vi "Main.vi"() -> ()   [LabVIEW 2021] (continued)
                    w1503 = T9 27 items=["刷新间隔", "波特率", "布尔1设置项", "布尔2设置项", "布尔3设置项", "布尔4设置项", "布尔5设置项", "布尔6设置项", "布尔7设置项", "布尔8设置项", "显控1设置", "显控2设置", "显控3设置", "显控4设置", "显控5设置", "显控6设置", "显控7设置", "显控8设置", "显控9设置", "显控10设置", "显控11设置", "显控12设置", "设控1设置", "设控2设置", "设控3设置", "设控4设置", "设控5设置", "设控6设置", "设控7设置", "设控8设置", "曲线1设置", "曲线2设置", "曲线3设置", "曲线4设置", "曲线5设置", "曲线6设置", "曲线7设置", "曲线8设置", "曲线9设置", "曲线10设置", "曲线11设置", "曲线12设置", "曲线13设置", "曲线14设置", "曲线15设置", "曲线16设置", "曲线17设置", "曲线18设置", "曲线19设置", "曲线20设置", "曲线21设置", "曲线22设置", "曲线23设置", "曲线24设置", "曲线25设置", "曲线26设置", "曲线27设置", "曲线28设置", "曲线29设置", "曲线30设置", "曲线31设置", "曲线32设置", "曲线33设置", "曲线34设置", "曲线35设置", "曲线36设置", "曲线37设置", "曲线38设置", "曲线39设置", "曲线40设置", "曲线41设置", "曲线42设置", "曲线43设置", "曲线44设置", "曲线45设置", "曲线46设置", "曲线47设置", "曲线48设置", "曲线49设置", "曲线50设置", "曲线51设置", "曲线52设置", "曲线53设置", "曲线54设置", "曲线55设置", "曲线56设置", "曲线57设置", "曲线58设置", "曲线59设置", "曲线60设置", "曲线61设置", "曲线62设置", "曲线63设置", "曲线64设置", "ID值", "数据模式"] ("DataInitDef")
                    n1213 = property on="表格" class="Tbl (严格)"() -> ("Selection Start"=w1510:T1)  [unwired: 2 in, 2 out]
                    n1214 = Unbundle By Name(w1510) -> ("Row"=w1512:i32)
                    n1215 = property on="表格" class="Tbl (严格)"() -> ("Value"=w1511:string[][])  [unwired: 2 in, 2 out]
                    n1216 = Number To Decimal String(number=w1512) -> (decimal integer string=w1513:string)  [unwired: 1 in]
                    n1217 = Index Array(array=w1511, index (row)=w1512, index (col)=0 ("禁用的索引 (列)")) -> (element=w1505:string)
                    n1218 = String Subset(string=w1505, length (rest)=16 ("长度（剩余）")) -> (substring=w1504:string)  [unwired: 1 in]
                    n1219 = invoke on="控件配置文件" class="Tbl (严格)" method="Set Cell Value"("X Index"=1 ("X索引"), "Y Index"=w1503, "Value"=w1513) -> ()  [unwired: 3 in, 6 out]
                    n1220 = property on="设控6" class="Str"("Caption.Text"=w1504) -> ()  [unwired: 2 in, 2 out]
                    n1221 = property on="设控设置 6" class="Str"("Val(Sgnl)"=w1504) -> ()  [unwired: 2 in, 2 out]
                    n1222 = invoke on="控件配置文件" class="Tbl (严格)" method="Set Cell Value"("X Index"=0 ("X索引"), "Y Index"=w1503, "Value"=w1504) -> ()  [unwired: 3 in, 6 out]
                  }
                  frame "关联到设控7" {
                    w1514 = T9 28 items=["刷新间隔", "波特率", "布尔1设置项", "布尔2设置项", "布尔3设置项", "布尔4设置项", "布尔5设置项", "布尔6设置项", "布尔7设置项", "布尔8设置项", "显控1设置", "显控2设置", "显控3设置", "显控4设置", "显控5设置", "显控6设置", "显控7设置", "显控8设置", "显控9设置", "显控10设置", "显控11设置", "显控12设置", "设控1设置", "设控2设置", "设控3设置", "设控4设置", "设控5设置", "设控6设置", "设控7设置", "设控8设置", "曲线1设置", "曲线2设置", "曲线3设置", "曲线4设置", "曲线5设置", "曲线6设置", "曲线7设置", "曲线8设置", "曲线9设置", "曲线10设置", "曲线11设置", "曲线12设置", "曲线13设置", "曲线14设置", "曲线15设置", "曲线16设置", "曲线17设置", "曲线18设置", "曲线19设置", "曲线20设置", "曲线21设置", "曲线22设置", "曲线23设置", "曲线24设置", "曲线25设置", "曲线26设置", "曲线27设置", "曲线28设置", "曲线29设置", "曲线30设置", "曲线31设置", "曲线32设置", "曲线33设置", "曲线34设置", "曲线35设置", "曲线36设置", "曲线37设置", "曲线38设置", "曲线39设置", "曲线40设置", "曲线41设置", "曲线42设置", "曲线43设置", "曲线44设置", "曲线45设置", "曲线46设置", "曲线47设置", "曲线48设置", "曲线49设置", "曲线50设置", "曲线51设置", "曲线52设置", "曲线53设置", "曲线54设置", "曲线55设置", "曲线56设置", "曲线57设置", "曲线58设置", "曲线59设置", "曲线60设置", "曲线61设置", "曲线62设置", "曲线63设置", "曲线64设置", "ID值", "数据模式"] ("DataInitDef")
                    n1223 = property on="表格" class="Tbl (严格)"() -> ("Selection Start"=w1524:T1)  [unwired: 2 in, 2 out]
                    n1224 = Unbundle By Name(w1524) -> ("Row"=w1522:i32)
                    n1225 = property on="表格" class="Tbl (严格)"() -> ("Value"=w1523:string[][])  [unwired: 2 in, 2 out]
                    n1226 = Number To Decimal String(number=w1522) -> (decimal integer string=w1521:string)  [unwired: 1 in]
                    n1227 = Index Array(array=w1523, index (row)=w1522, index (col)=0 ("禁用的索引 (列)")) -> (element=w1516:string)
                    n1228 = String Subset(string=w1516, length (rest)=16 ("长度（剩余）")) -> (substring=w1515:string)  [unwired: 1 in]
                    n1229 = invoke on="控件配置文件" class="Tbl (严格)" method="Set Cell Value"("X Index"=1 ("X索引"), "Y Index"=w1514, "Value"=w1521) -> ()  [unwired: 3 in, 6 out]
                    n1230 = property on="设控7" class="Str"("Caption.Text"=w1515) -> ()  [unwired: 2 in, 2 out]
                    n1231 = property on="设控设置 7" class="Str"("Val(Sgnl)"=w1515) -> ()  [unwired: 2 in, 2 out]
                    n1232 = invoke on="控件配置文件" class="Tbl (严格)" method="Set Cell Value"("X Index"=0 ("X索引"), "Y Index"=w1514, "Value"=w1515) -> ()  [unwired: 3 in, 6 out]
                  }
                  frame "关联到设控8" {
                    w1525 = T9 29 items=["刷新间隔", "波特率", "布尔1设置项", "布尔2设置项", "布尔3设置项", "布尔4设置项", "布尔5设置项", "布尔6设置项", "布尔7设置项", "布尔8设置项", "显控1设置", "显控2设置", "显控3设置", "显控4设置", "显控5设置", "显控6设置", "显控7设置", "显控8设置", "显控9设置", "显控10设置", "显控11设置", "显控12设置", "设控1设置", "设控2设置", "设控3设置", "设控4设置", "设控5设置", "设控6设置", "设控7设置", "设控8设置", "曲线1设置", "曲线2设置", "曲线3设置", "曲线4设置", "曲线5设置", "曲线6设置", "曲线7设置", "曲线8设置", "曲线9设置", "曲线10设置", "曲线11设置", "曲线12设置", "曲线13设置", "曲线14设置", "曲线15设置", "曲线16设置", "曲线17设置", "曲线18设置", "曲线19设置", "曲线20设置", "曲线21设置", "曲线22设置", "曲线23设置", "曲线24设置", "曲线25设置", "曲线26设置", "曲线27设置", "曲线28设置", "曲线29设置", "曲线30设置", "曲线31设置", "曲线32设置", "曲线33设置", "曲线34设置", "曲线35设置", "曲线36设置", "曲线37设置", "曲线38设置", "曲线39设置", "曲线40设置", "曲线41设置", "曲线42设置", "曲线43设置", "曲线44设置", "曲线45设置", "曲线46设置", "曲线47设置", "曲线48设置", "曲线49设置", "曲线50设置", "曲线51设置", "曲线52设置", "曲线53设置", "曲线54设置", "曲线55设置", "曲线56设置", "曲线57设置", "曲线58设置", "曲线59设置", "曲线60设置", "曲线61设置", "曲线62设置", "曲线63设置", "曲线64设置", "ID值", "数据模式"] ("DataInitDef")
                    n1233 = property on="表格" class="Tbl (严格)"() -> ("Selection Start"=w1532:T1)  [unwired: 2 in, 2 out]
                    n1234 = Unbundle By Name(w1532) -> ("Row"=w1534:i32)
                    n1235 = property on="表格" class="Tbl (严格)"() -> ("Value"=w1533:string[][])  [unwired: 2 in, 2 out]
                    n1236 = Number To Decimal String(number=w1534) -> (decimal integer string=w1535:string)  [unwired: 1 in]
                    n1237 = Index Array(array=w1533, index (row)=w1534, index (col)=0 ("禁用的索引 (列)")) -> (element=w1527:string)
                    n1238 = String Subset(string=w1527, length (rest)=16 ("长度（剩余）")) -> (substring=w1526:string)  [unwired: 1 in]
                    n1239 = invoke on="控件配置文件" class="Tbl (严格)" method="Set Cell Value"("X Index"=1 ("X索引"), "Y Index"=w1525, "Value"=w1535) -> ()  [unwired: 3 in, 6 out]
                    n1240 = property on="设控8" class="Str"("Caption.Text"=w1526) -> ()  [unwired: 2 in, 2 out]
                    n1241 = property on="设控设置 8" class="Str"("Val(Sgnl)"=w1526) -> ()  [unwired: 2 in, 2 out]
                    n1242 = invoke on="控件配置文件" class="Tbl (严格)" method="Set Cell Value"("X Index"=0 ("X索引"), "Y Index"=w1525, "Value"=w1526) -> ()  [unwired: 3 in, 6 out]
                  }
                }
              }
            }
          }
          frame #2 {
            # "快捷菜单激活何批量EEPROM、数据导出"
            n1243 = event shown="[1] 菜单选择(用户);  \"表格\": 快捷菜单选择（用户）" {
              selector: _ -> [_ _]
              dyn-events: _ -> [_ _]
              timeout: 0 -> [_ _]
              event Timeout {
                n1244 = event-data() -> ()  [unwired: 1 in, 3 out]
              }
              event Menu Selection (User); "表格": Shortcut Menu Selection (User) {
                n1245 = event-data() -> ("ItemTag"=w1549:string)  [unwired: 1 in, 5 out]
                n1246 = case shown="\"批量写入EEPROM\"" w1549 {
                  frame "假", Default {
                  }
                  frame "导出参数" {
                    n1247 = property on="表格" class="Tbl (严格)"() -> ("Value"=w1552:string[][])  [unwired: 2 in, 2 out]
                    n1248 = call <vilib>:"Application Directory.vi"() -> ("Application Directory"=w1551:path)
                    n1249 = call "导出参数.vi"("名称或相对路径"="Config\\导出参数列表.xltx", "基路径"=w1551, "表格控件"=w1552) -> ()  [unwired: 9 in]
                  }
                  frame "批量写入EEPROM" {
                    n1250 = local read "刷新间隔"() -> (w1559:string)
                    n1251 = Decimal String To Number(string=w1559) -> (number=w1557:i32)  [unwired: 2 in, 1 out]
                    n1252 = local read "CAN通道"() -> (w1553:u8)
                    n1253 = local read "ID"() -> (w1554:u32)
                    n1254 = Less Or Equal?(x=w1557, y=1) -> (x <= y?=w1555:bool)
                    n1255 = Select(t=1, s=w1555, f=w1557) -> (s? t:f=w1558:i32)
                    n1256 = call "批量写入EEPROM.vi"("等待时间（毫秒）"=w1558, "ID"=w1554, "CAN通道"=w1553) -> ()  [unwired: 8 in]
                  }
                }
              }
            }
            n1257 = event shown="[1] \"波形图表\": 快捷菜单激活？" {
              selector: _ -> [_ _]
              dyn-events: _ -> [_ _]
              timeout: 0 -> [_ _]
              event Timeout {
                n1258 = event-data() -> ()  [unwired: 1 in, 3 out]
              }
              event "波形图表": Shortcut Menu Activation? {
                n1259 = event-data() -> ("MenuRef"=w1548:refnum<k9>)  [unwired: 1 in]
                n1260 = call "快捷菜单激活(波形图表).vi"("菜单引用"=w1548) -> ()  [unwired: 11 in]
                n1261 = event-data() -> ()  [unwired: 2 in, 1 out]
              }
            }
            n1262 = event shown="[1] \"表格\": 快捷菜单激活？" {
              selector: _ -> [_ _]
              dyn-events: _ -> [_ _]
              timeout: 0 -> [_ _]
              event Timeout {
                n1263 = event-data() -> ()  [unwired: 1 in, 3 out]
              }
              event "表格": Shortcut Menu Activation? {
                # "激活表格右击菜单选项"
                n1264 = event-data() -> ("MenuRef"=w1561:refnum<k9>)  [unwired: 1 in]
                n1265 = call "快捷菜单激活(表格).vi"("菜单引用"=w1561) -> ()  [unwired: 11 in]
                n1266 = event-data() -> ()  [unwired: 2 in, 1 out]
              }
            }
            n1267 = event shown="[1] \"布尔 1\", \"布尔 2\", \"布尔 3\", \"布尔 4\", \"布尔 5\", \"布尔 6\", \"布尔 7\", \"布尔 8\": 快捷菜单激活？" {
              selector: _ -> [_ _ _ _ _]
              dyn-events: _ -> [_ _ _ _ _]
              timeout: 0 -> [_ _ _ _ _]
              event Timeout {
                n1268 = event-data() -> ()  [unwired: 1 in, 3 out]
              }
              event "布尔 1", "布尔 2", "布尔 3", "布尔 4", "布尔 5", "布尔 6", "布尔 7", "布尔 8": Shortcut Menu Activation? {
                # "撤销布尔控件的关联"
                n1269 = event-data() -> ("MenuRef"=w1541:refnum<k9>)  [unwired: 1 in, 3 out]
                n1270 = Insert Menu Items(8:string[] ["撤销关联"] ("项名称"), 9:w1541) -> ()  [unwired: 4 in, 3 out]
                n1271 = event-data() -> ()  [unwired: 2 in, 1 out]
              }
              event "显控1", "显控6", "显控7", "显控2", "显控3", "显控4", "显控8", "显控9", "显控10", "显控11", "显控12", "显控5": Shortcut Menu Activation? {
                n1272 = event-data() -> ("MenuRef"=w1542:refnum<k9>)  [unwired: 1 in, 4 out]
                n1273 = Insert Menu Items(8:string[] ["撤销关联"] ("项名称"), 9:w1542) -> ()  [unwired: 4 in, 3 out]
                n1274 = event-data() -> ()  [unwired: 2 in, 1 out]
              }
              event "设控1", "设控2", "设控3", "设控4", "设控5", "设控6", "设控7", "设控8": Shortcut Menu Activation? {
                n1275 = event-data() -> ("MenuRef"=w1544:refnum<k9>)  [unwired: 1 in, 5 out]
                n1276 = event-data() -> ()  [unwired: 2 in, 1 out]
                n1277 = Insert Menu Items(8:string[] ["撤销关联"] ("项名称"), 9:w1544) -> ()  [unwired: 4 in, 3 out]
              }
              event "状态显示": Shortcut Menu Activation? {
                n1278 = event-data() -> ("MenuRef"=w1546:refnum<k9>)  [unwired: 1 in, 5 out]
                n1279 = event-data() -> ()  [unwired: 2 in, 1 out]
                n1280 = Insert Menu Items(8:string[] ["撤销关联"] ("项名称"), 9:w1546) -> ()  [unwired: 4 in, 3 out]
              }
            }
          }
          frame #3 {
            # "所有控件撤销关联代码"
            n1281 = event shown="[21] \"波形图表\": 快捷菜单选择（用户）" {
              selector: _ -> [_ _ _ _ _ _ _ _ _ _ _ _ _ _ _ _ _ _ _ _ _ _ _ _ _ _ _ _ _ _]
              dyn-events: _ -> [_ _ _ _ _ _ _ _ _ _ _ _ _ _ _ _ _ _ _ _ _ _ _ _ _ _ _ _ _ _]
              timeout: 0 -> [_ _ _ _ _ _ _ _ _ _ _ _ _ _ _ _ _ _ _ _ _ _ _ _ _ _ _ _ _ _]
              event Timeout {
                n1282 = event-data() -> ()  [unwired: 1 in, 3 out]
              }
              event "布尔 1": Shortcut Menu Selection (User) {
                w1563 = T9 2 items=["刷新间隔", "波特率", "布尔1设置项", "布尔2设置项", "布尔3设置项", "布尔4设置项", "布尔5设置项", "布尔6设置项", "布尔7设置项", "布尔8设置项", "显控1设置", "显控2设置", "显控3设置", "显控4设置", "显控5设置", "显控6设置", "显控7设置", "显控8设置", "显控9设置", "显控10设置", "显控11设置", "显控12设置", "设控1设置", "设控2设置", "设控3设置", "设控4设置", "设控5设置", "设控6设置", "设控7设置", "设控8设置", "曲线1设置", "曲线2设置", "曲线3设置", "曲线4设置", "曲线5设置", "曲线6设置", "曲线7设置", "曲线8设置", "曲线9设置", "曲线10设置", "曲线11设置", "曲线12设置", "曲线13设置", "曲线14设置", "曲线15设置", "曲线16设置", "曲线17设置", "曲线18设置", "曲线19设置", "曲线20设置", "曲线21设置", "曲线22设置", "曲线23设置", "曲线24设置", "曲线25设置", "曲线26设置", "曲线27设置", "曲线28设置", "曲线29设置", "曲线30设置", "曲线31设置", "曲线32设置", "曲线33设置", "曲线34设置", "曲线35设置", "曲线36设置", "曲线37设置", "曲线38设置", "曲线39设置", "曲线40设置", "曲线41设置", "曲线42设置", "曲线43设置", "曲线44设置", "曲线45设置", "曲线46设置", "曲线47设置", "曲线48设置", "曲线49设置", "曲线50设置", "曲线51设置", "曲线52设置", "曲线53设置", "曲线54设置", "曲线55设置", "曲线56设置", "曲线57设置", "曲线58设置", "曲线59设置", "曲线60设置", "曲线61设置", "曲线62设置", "曲线63设置", "曲线64设置", "ID值", "数据模式"] ("DataInitDef")
                w1564 = "布尔 1" ("标题.文本")
                # "撤销关联的代码"
                n1283 = event-data() -> ()  [unwired: 1 in, 8 out]
                n1284 = invoke on="控件配置文件" class="Tbl (严格)" method="Set Cell Value"("X Index"=1 ("X索引"), "Y Index"=w1563, "Value"="X" ("值")) -> ()  [unwired: 3 in, 6 out]
                n1285 = invoke on="控件配置文件" class="Tbl (严格)" method="Set Cell Value"("X Index"=0 ("X索引"), "Y Index"=w1563, "Value"=w1564) -> ()  [unwired: 3 in, 6 out]
                n1286 = property on="布尔 1" class="Bool (严格)"("Caption.Text"=w1564) -> ()  [unwired: 2 in, 2 out]
                n1287 = property on="布控1设置" class="Str"("Val(Sgnl)"=w1564) -> ()  [unwired: 2 in, 2 out]
              }
              event "布尔 2": Shortcut Menu Selection (User) {
                w1568 = T9 3 items=["刷新间隔", "波特率", "布尔1设置项", "布尔2设置项", "布尔3设置项", "布尔4设置项", "布尔5设置项", "布尔6设置项", "布尔7设置项", "布尔8设置项", "显控1设置", "显控2设置", "显控3设置", "显控4设置", "显控5设置", "显控6设置", "显控7设置", "显控8设置", "显控9设置", "显控10设置", "显控11设置", "显控12设置", "设控1设置", "设控2设置", "设控3设置", "设控4设置", "设控5设置", "设控6设置", "设控7设置", "设控8设置", "曲线1设置", "曲线2设置", "曲线3设置", "曲线4设置", "曲线5设置", "曲线6设置", "曲线7设置", "曲线8设置", "曲线9设置", "曲线10设置", "曲线11设置", "曲线12设置", "曲线13设置", "曲线14设置", "曲线15设置", "曲线16设置", "曲线17设置", "曲线18设置", "曲线19设置", "曲线20设置", "曲线21设置", "曲线22设置", "曲线23设置", "曲线24设置", "曲线25设置", "曲线26设置", "曲线27设置", "曲线28设置", "曲线29设置", "曲线30设置", "曲线31设置", "曲线32设置", "曲线33设置", "曲线34设置", "曲线35设置", "曲线36设置", "曲线37设置", "曲线38设置", "曲线39设置", "曲线40设置", "曲线41设置", "曲线42设置", "曲线43设置", "曲线44设置", "曲线45设置", "曲线46设置", "曲线47设置", "曲线48设置", "曲线49设置", "曲线50设置", "曲线51设置", "曲线52设置", "曲线53设置", "曲线54设置", "曲线55设置", "曲线56设置", "曲线57设置", "曲线58设置", "曲线59设置", "曲线60设置", "曲线61设置", "曲线62设置", "曲线63设置", "曲线64设置", "ID值", "数据模式"] ("DataInitDef")
                w1569 = "布尔 2" ("标题.文本")
                n1288 = event-data() -> ()  [unwired: 1 in, 8 out]
                n1289 = invoke on="控件配置文件" class="Tbl (严格)" method="Set Cell Value"("X Index"=1 ("X索引"), "Y Index"=w1568, "Value"="X" ("值")) -> ()  [unwired: 3 in, 6 out]
                n1290 = invoke on="控件配置文件" class="Tbl (严格)" method="Set Cell Value"("X Index"=0 ("X索引"), "Y Index"=w1568, "Value"=w1569) -> ()  [unwired: 3 in, 6 out]
                n1291 = property on="布控2设置" class="Str"("Val(Sgnl)"=w1569) -> ()  [unwired: 2 in, 2 out]
                n1292 = property on="布尔 2" class="Bool (严格)"("Caption.Text"=w1569) -> ()  [unwired: 2 in, 2 out]
              }
              event "布尔 3": Shortcut Menu Selection (User) {
                w1573 = T9 4 items=["刷新间隔", "波特率", "布尔1设置项", "布尔2设置项", "布尔3设置项", "布尔4设置项", "布尔5设置项", "布尔6设置项", "布尔7设置项", "布尔8设置项", "显控1设置", "显控2设置", "显控3设置", "显控4设置", "显控5设置", "显控6设置", "显控7设置", "显控8设置", "显控9设置", "显控10设置", "显控11设置", "显控12设置", "设控1设置", "设控2设置", "设控3设置", "设控4设置", "设控5设置", "设控6设置", "设控7设置", "设控8设置", "曲线1设置", "曲线2设置", "曲线3设置", "曲线4设置", "曲线5设置", "曲线6设置", "曲线7设置", "曲线8设置", "曲线9设置", "曲线10设置", "曲线11设置", "曲线12设置", "曲线13设置", "曲线14设置", "曲线15设置", "曲线16设置", "曲线17设置", "曲线18设置", "曲线19设置", "曲线20设置", "曲线21设置", "曲线22设置", "曲线23设置", "曲线24设置", "曲线25设置", "曲线26设置", "曲线27设置", "曲线28设置", "曲线29设置", "曲线30设置", "曲线31设置", "曲线32设置", "曲线33设置", "曲线34设置", "曲线35设置", "曲线36设置", "曲线37设置", "曲线38设置", "曲线39设置", "曲线40设置", "曲线41设置", "曲线42设置", "曲线43设置", "曲线44设置", "曲线45设置", "曲线46设置", "曲线47设置", "曲线48设置", "曲线49设置", "曲线50设置", "曲线51设置", "曲线52设置", "曲线53设置", "曲线54设置", "曲线55设置", "曲线56设置", "曲线57设置", "曲线58设置", "曲线59设置", "曲线60设置", "曲线61设置", "曲线62设置", "曲线63设置", "曲线64设置", "ID值", "数据模式"] ("DataInitDef")
                w1574 = "布尔 3" ("标题.文本")
                n1293 = event-data() -> ()  [unwired: 1 in, 8 out]
                n1294 = invoke on="控件配置文件" class="Tbl (严格)" method="Set Cell Value"("X Index"=1 ("X索引"), "Y Index"=w1573, "Value"="X" ("值")) -> ()  [unwired: 3 in, 6 out]
                n1295 = invoke on="控件配置文件" class="Tbl (严格)" method="Set Cell Value"("X Index"=0 ("X索引"), "Y Index"=w1573, "Value"=w1574) -> ()  [unwired: 3 in, 6 out]
                n1296 = property on="布尔 3" class="Bool (严格)"("Caption.Text"=w1574) -> ()  [unwired: 2 in, 2 out]
                n1297 = property on="布控3设置" class="Str"("Val(Sgnl)"=w1574) -> ()  [unwired: 2 in, 2 out]
              }
              event "布尔 4": Shortcut Menu Selection (User) {
                w1578 = T9 5 items=["刷新间隔", "波特率", "布尔1设置项", "布尔2设置项", "布尔3设置项", "布尔4设置项", "布尔5设置项", "布尔6设置项", "布尔7设置项", "布尔8设置项", "显控1设置", "显控2设置", "显控3设置", "显控4设置", "显控5设置", "显控6设置", "显控7设置", "显控8设置", "显控9设置", "显控10设置", "显控11设置", "显控12设置", "设控1设置", "设控2设置", "设控3设置", "设控4设置", "设控5设置", "设控6设置", "设控7设置", "设控8设置", "曲线1设置", "曲线2设置", "曲线3设置", "曲线4设置", "曲线5设置", "曲线6设置", "曲线7设置", "曲线8设置", "曲线9设置", "曲线10设置", "曲线11设置", "曲线12设置", "曲线13设置", "曲线14设置", "曲线15设置", "曲线16设置", "曲线17设置", "曲线18设置", "曲线19设置", "曲线20设置", "曲线21设置", "曲线22设置", "曲线23设置", "曲线24设置", "曲线25设置", "曲线26设置", "曲线27设置", "曲线28设置", "曲线29设置", "曲线30设置", "曲线31设置", "曲线32设置", "曲线33设置", "曲线34设置", "曲线35设置", "曲线36设置", "曲线37设置", "曲线38设置", "曲线39设置", "曲线40设置", "曲线41设置", "曲线42设置", "曲线43设置", "曲线44设置", "曲线45设置", "曲线46设置", "曲线47设置", "曲线48设置", "曲线49设置", "曲线50设置", "曲线51设置", "曲线52设置", "曲线53设置", "曲线54设置", "曲线55设置", "曲线56设置", "曲线57设置", "曲线58设置", "曲线59设置", "曲线60设置", "曲线61设置", "曲线62设置", "曲线63设置", "曲线64设置", "ID值", "数据模式"] ("DataInitDef")
                w1579 = "布尔 4" ("标题.文本")
                n1298 = event-data() -> ()  [unwired: 1 in, 8 out]
                n1299 = invoke on="控件配置文件" class="Tbl (严格)" method="Set Cell Value"("X Index"=1 ("X索引"), "Y Index"=w1578, "Value"="X" ("值")) -> ()  [unwired: 3 in, 6 out]
                n1300 = invoke on="控件配置文件" class="Tbl (严格)" method="Set Cell Value"("X Index"=0 ("X索引"), "Y Index"=w1578, "Value"=w1579) -> ()  [unwired: 3 in, 6 out]
                n1301 = property on="布尔 4" class="Bool (严格)"("Caption.Text"=w1579) -> ()  [unwired: 2 in, 2 out]
                n1302 = property on="布控4设置" class="Str"("Val(Sgnl)"=w1579) -> ()  [unwired: 2 in, 2 out]
              }
              event "布尔 5": Shortcut Menu Selection (User) {
                w1583 = T9 6 items=["刷新间隔", "波特率", "布尔1设置项", "布尔2设置项", "布尔3设置项", "布尔4设置项", "布尔5设置项", "布尔6设置项", "布尔7设置项", "布尔8设置项", "显控1设置", "显控2设置", "显控3设置", "显控4设置", "显控5设置", "显控6设置", "显控7设置", "显控8设置", "显控9设置", "显控10设置", "显控11设置", "显控12设置", "设控1设置", "设控2设置", "设控3设置", "设控4设置", "设控5设置", "设控6设置", "设控7设置", "设控8设置", "曲线1设置", "曲线2设置", "曲线3设置", "曲线4设置", "曲线5设置", "曲线6设置", "曲线7设置", "曲线8设置", "曲线9设置", "曲线10设置", "曲线11设置", "曲线12设置", "曲线13设置", "曲线14设置", "曲线15设置", "曲线16设置", "曲线17设置", "曲线18设置", "曲线19设置", "曲线20设置", "曲线21设置", "曲线22设置", "曲线23设置", "曲线24设置", "曲线25设置", "曲线26设置", "曲线27设置", "曲线28设置", "曲线29设置", "曲线30设置", "曲线31设置", "曲线32设置", "曲线33设置", "曲线34设置", "曲线35设置", "曲线36设置", "曲线37设置", "曲线38设置", "曲线39设置", "曲线40设置", "曲线41设置", "曲线42设置", "曲线43设置", "曲线44设置", "曲线45设置", "曲线46设置", "曲线47设置", "曲线48设置", "曲线49设置", "曲线50设置", "曲线51设置", "曲线52设置", "曲线53设置", "曲线54设置", "曲线55设置", "曲线56设置", "曲线57设置", "曲线58设置", "曲线59设置", "曲线60设置", "曲线61设置", "曲线62设置", "曲线63设置", "曲线64设置", "ID值", "数据模式"] ("DataInitDef")
                w1587 = "布尔 5" ("标题.文本")
                n1303 = event-data() -> ()  [unwired: 1 in, 8 out]
                n1304 = invoke on="控件配置文件" class="Tbl (严格)" method="Set Cell Value"("X Index"=1 ("X索引"), "Y Index"=w1583, "Value"="X" ("值")) -> ()  [unwired: 3 in, 6 out]
                n1305 = invoke on="控件配置文件" class="Tbl (严格)" method="Set Cell Value"("X Index"=0 ("X索引"), "Y Index"=w1583, "Value"=w1587) -> ()  [unwired: 3 in, 6 out]
                n1306 = property on="布尔 5" class="Bool (严格)"("Caption.Text"=w1587) -> ()  [unwired: 2 in, 2 out]
                n1307 = property on="布控5设置" class="Str"("Val(Sgnl)"=w1587) -> ()  [unwired: 2 in, 2 out]
              }
              event "布尔 6": Shortcut Menu Selection (User) {
                w1590 = T9 7 items=["刷新间隔", "波特率", "布尔1设置项", "布尔2设置项", "布尔3设置项", "布尔4设置项", "布尔5设置项", "布尔6设置项", "布尔7设置项", "布尔8设置项", "显控1设置", "显控2设置", "显控3设置", "显控4设置", "显控5设置", "显控6设置", "显控7设置", "显控8设置", "显控9设置", "显控10设置", "显控11设置", "显控12设置", "设控1设置", "设控2设置", "设控3设置", "设控4设置", "设控5设置", "设控6设置", "设控7设置", "设控8设置", "曲线1设置", "曲线2设置", "曲线3设置", "曲线4设置", "曲线5设置", "曲线6设置", "曲线7设置", "曲线8设置", "曲线9设置", "曲线10设置", "曲线11设置", "曲线12设置", "曲线13设置", "曲线14设置", "曲线15设置", "曲线16设置", "曲线17设置", "曲线18设置", "曲线19设置", "曲线20设置", "曲线21设置", "曲线22设置", "曲线23设置", "曲线24设置", "曲线25设置", "曲线26设置", "曲线27设置", "曲线28设置", "曲线29设置", "曲线30设置", "曲线31设置", "曲线32设置", "曲线33设置", "曲线34设置", "曲线35设置", "曲线36设置", "曲线37设置", "曲线38设置", "曲线39设置", "曲线40设置", "曲线41设置", "曲线42设置", "曲线43设置", "曲线44设置", "曲线45设置", "曲线46设置", "曲线47设置", "曲线48设置", "曲线49设置", "曲线50设置", "曲线51设置", "曲线52设置", "曲线53设置", "曲线54设置", "曲线55设置", "曲线56设置", "曲线57设置", "曲线58设置", "曲线59设置", "曲线60设置", "曲线61设置", "曲线62设置", "曲线63设置", "曲线64设置", "ID值", "数据模式"] ("DataInitDef")
                w1592 = "布尔 6" ("标题.文本")
                n1308 = event-data() -> ()  [unwired: 1 in, 8 out]
                n1309 = invoke on="控件配置文件" class="Tbl (严格)" method="Set Cell Value"("X Index"=1 ("X索引"), "Y Index"=w1590, "Value"="X" ("值")) -> ()  [unwired: 3 in, 6 out]
                n1310 = invoke on="控件配置文件" class="Tbl (严格)" method="Set Cell Value"("X Index"=0 ("X索引"), "Y Index"=w1590, "Value"=w1592) -> ()  [unwired: 3 in, 6 out]
                n1311 = property on="布尔 6" class="Bool (严格)"("Caption.Text"=w1592) -> ()  [unwired: 2 in, 2 out]
                n1312 = property on="布控6设置" class="Str"("Val(Sgnl)"=w1592) -> ()  [unwired: 2 in, 2 out]
              }
              event "布尔 7": Shortcut Menu Selection (User) {
                w1595 = T9 8 items=["刷新间隔", "波特率", "布尔1设置项", "布尔2设置项", "布尔3设置项", "布尔4设置项", "布尔5设置项", "布尔6设置项", "布尔7设置项", "布尔8设置项", "显控1设置", "显控2设置", "显控3设置", "显控4设置", "显控5设置", "显控6设置", "显控7设置", "显控8设置", "显控9设置", "显控10设置", "显控11设置", "显控12设置", "设控1设置", "设控2设置", "设控3设置", "设控4设置", "设控5设置", "设控6设置", "设控7设置", "设控8设置", "曲线1设置", "曲线2设置", "曲线3设置", "曲线4设置", "曲线5设置", "曲线6设置", "曲线7设置", "曲线8设置", "曲线9设置", "曲线10设置", "曲线11设置", "曲线12设置", "曲线13设置", "曲线14设置", "曲线15设置", "曲线16设置", "曲线17设置", "曲线18设置", "曲线19设置", "曲线20设置", "曲线21设置", "曲线22设置", "曲线23设置", "曲线24设置", "曲线25设置", "曲线26设置", "曲线27设置", "曲线28设置", "曲线29设置", "曲线30设置", "曲线31设置", "曲线32设置", "曲线33设置", "曲线34设置", "曲线35设置", "曲线36设置", "曲线37设置", "曲线38设置", "曲线39设置", "曲线40设置", "曲线41设置", "曲线42设置", "曲线43设置", "曲线44设置", "曲线45设置", "曲线46设置", "曲线47设置", "曲线48设置", "曲线49设置", "曲线50设置", "曲线51设置", "曲线52设置", "曲线53设置", "曲线54设置", "曲线55设置", "曲线56设置", "曲线57设置", "曲线58设置", "曲线59设置", "曲线60设置", "曲线61设置", "曲线62设置", "曲线63设置", "曲线64设置", "ID值", "数据模式"] ("DataInitDef")
                w1597 = "布尔 7" ("标题.文本")
                n1313 = event-data() -> ()  [unwired: 1 in, 8 out]
                n1314 = invoke on="控件配置文件" class="Tbl (严格)" method="Set Cell Value"("X Index"=1 ("X索引"), "Y Index"=w1595, "Value"="X" ("值")) -> ()  [unwired: 3 in, 6 out]
                n1315 = invoke on="控件配置文件" class="Tbl (严格)" method="Set Cell Value"("X Index"=0 ("X索引"), "Y Index"=w1595, "Value"=w1597) -> ()  [unwired: 3 in, 6 out]
                n1316 = property on="布尔 7" class="Bool (严格)"("Caption.Text"=w1597) -> ()  [unwired: 2 in, 2 out]
                n1317 = property on="布控7设置" class="Str"("Val(Sgnl)"=w1597) -> ()  [unwired: 2 in, 2 out]
              }
              event "布尔 8": Shortcut Menu Selection (User) {
                w1600 = T9 9 items=["刷新间隔", "波特率", "布尔1设置项", "布尔2设置项", "布尔3设置项", "布尔4设置项", "布尔5设置项", "布尔6设置项", "布尔7设置项", "布尔8设置项", "显控1设置", "显控2设置", "显控3设置", "显控4设置", "显控5设置", "显控6设置", "显控7设置", "显控8设置", "显控9设置", "显控10设置", "显控11设置", "显控12设置", "设控1设置", "设控2设置", "设控3设置", "设控4设置", "设控5设置", "设控6设置", "设控7设置", "设控8设置", "曲线1设置", "曲线2设置", "曲线3设置", "曲线4设置", "曲线5设置", "曲线6设置", "曲线7设置", "曲线8设置", "曲线9设置", "曲线10设置", "曲线11设置", "曲线12设置", "曲线13设置", "曲线14设置", "曲线15设置", "曲线16设置", "曲线17设置", "曲线18设置", "曲线19设置", "曲线20设置", "曲线21设置", "曲线22设置", "曲线23设置", "曲线24设置", "曲线25设置", "曲线26设置", "曲线27设置", "曲线28设置", "曲线29设置", "曲线30设置", "曲线31设置", "曲线32设置", "曲线33设置", "曲线34设置", "曲线35设置", "曲线36设置", "曲线37设置", "曲线38设置", "曲线39设置", "曲线40设置", "曲线41设置", "曲线42设置", "曲线43设置", "曲线44设置", "曲线45设置", "曲线46设置", "曲线47设置", "曲线48设置", "曲线49设置", "曲线50设置", "曲线51设置", "曲线52设置", "曲线53设置", "曲线54设置", "曲线55设置", "曲线56设置", "曲线57设置", "曲线58设置", "曲线59设置", "曲线60设置", "曲线61设置", "曲线62设置", "曲线63设置", "曲线64设置", "ID值", "数据模式"] ("DataInitDef")
                w1602 = "布尔 8" ("标题.文本")
                n1318 = event-data() -> ()  [unwired: 1 in, 8 out]
                n1319 = invoke on="控件配置文件" class="Tbl (严格)" method="Set Cell Value"("X Index"=1 ("X索引"), "Y Index"=w1600, "Value"="X" ("值")) -> ()  [unwired: 3 in, 6 out]
                n1320 = invoke on="控件配置文件" class="Tbl (严格)" method="Set Cell Value"("X Index"=0 ("X索引"), "Y Index"=w1600, "Value"=w1602) -> ()  [unwired: 3 in, 6 out]
                n1321 = property on="布尔 8" class="Bool (严格)"("Caption.Text"=w1602) -> ()  [unwired: 2 in, 2 out]
                n1322 = property on="布控8设置" class="Str"("Val(Sgnl)"=w1602) -> ()  [unwired: 2 in, 2 out]
              }
              event "显控1": Shortcut Menu Selection (User) {
                w1603 = T9 10 items=["刷新间隔", "波特率", "布尔1设置项", "布尔2设置项", "布尔3设置项", "布尔4设置项", "布尔5设置项", "布尔6设置项", "布尔7设置项", "布尔8设置项", "显控1设置", "显控2设置", "显控3设置", "显控4设置", "显控5设置", "显控6设置", "显控7设置", "显控8设置", "显控9设置", "显控10设置", "显控11设置", "显控12设置", "设控1设置", "设控2设置", "设控3设置", "设控4设置", "设控5设置", "设控6设置", "设控7设置", "设控8设置", "曲线1设置", "曲线2设置", "曲线3设置", "曲线4设置", "曲线5设置", "曲线6设置", "曲线7设置", "曲线8设置", "曲线9设置", "曲线10设置", "曲线11设置", "曲线12设置", "曲线13设置", "曲线14设置", "曲线15设置", "曲线16设置", "曲线17设置", "曲线18设置", "曲线19设置", "曲线20设置", "曲线21设置", "曲线22设置", "曲线23设置", "曲线24设置", "曲线25设置", "曲线26设置", "曲线27设置", "曲线28设置", "曲线29设置", "曲线30设置", "曲线31设置", "曲线32设置", "曲线33设置", "曲线34设置", "曲线35设置", "曲线36设置", "曲线37设置", "曲线38设置", "曲线39设置", "曲线40设置", "曲线41设置", "曲线42设置", "曲线43设置", "曲线44设置", "曲线45设置", "曲线46设置", "曲线47设置", "曲线48设置", "曲线49设置", "曲线50设置", "曲线51设置", "曲线52设置", "曲线53设置", "曲线54设置", "曲线55设置", "曲线56设置", "曲线57设置", "曲线58设置", "曲线59设置", "曲线60设置", "曲线61设置", "曲线62设置", "曲线63设置", "曲线64设置", "ID值", "数据模式"] ("DataInitDef")
                w1604 = "显控1" ("标题.文本")
                # "撤销显控关联"
                n1323 = event-data() -> ()  [unwired: 1 in, 8 out]
                n1324 = invoke on="控件配置文件" class="Tbl (严格)" method="Set Cell Value"("X Index"=1 ("X索引"), "Y Index"=w1603, "Value"="X" ("值")) -> ()  [unwired: 3 in, 6 out]
                n1325 = invoke on="控件配置文件" class="Tbl (严格)" method="Set Cell Value"("X Index"=0 ("X索引"), "Y Index"=w1603, "Value"=w1604) -> ()  [unwired: 3 in, 6 out]
                n1326 = property on="显控1" class="Str"("Caption.Text"=w1604) -> ()  [unwired: 2 in, 2 out]
                n1327 = property on="显控1设置" class="Str"("Val(Sgnl)"=w1604) -> ()  [unwired: 2 in, 2 out]
              }
              event "显控2": Shortcut Menu Selection (User) {
                w1608 = T9 11 items=["刷新间隔", "波特率", "布尔1设置项", "布尔2设置项", "布尔3设置项", "布尔4设置项", "布尔5设置项", "布尔6设置项", "布尔7设置项", "布尔8设置项", "显控1设置", "显控2设置", "显控3设置", "显控4设置", "显控5设置", "显控6设置", "显控7设置", "显控8设置", "显控9设置", "显控10设置", "显控11设置", "显控12设置", "设控1设置", "设控2设置", "设控3设置", "设控4设置", "设控5设置", "设控6设置", "设控7设置", "设控8设置", "曲线1设置", "曲线2设置", "曲线3设置", "曲线4设置", "曲线5设置", "曲线6设置", "曲线7设置", "曲线8设置", "曲线9设置", "曲线10设置", "曲线11设置", "曲线12设置", "曲线13设置", "曲线14设置", "曲线15设置", "曲线16设置", "曲线17设置", "曲线18设置", "曲线19设置", "曲线20设置", "曲线21设置", "曲线22设置", "曲线23设置", "曲线24设置", "曲线25设置", "曲线26设置", "曲线27设置", "曲线28设置", "曲线29设置", "曲线30设置", "曲线31设置", "曲线32设置", "曲线33设置", "曲线34设置", "曲线35设置", "曲线36设置", "曲线37设置", "曲线38设置", "曲线39设置", "曲线40设置", "曲线41设置", "曲线42设置", "曲线43设置", "曲线44设置", "曲线45设置", "曲线46设置", "曲线47设置", "曲线48设置", "曲线49设置", "曲线50设置", "曲线51设置", "曲线52设置", "曲线53设置", "曲线54设置", "曲线55设置", "曲线56设置", "曲线57设置", "曲线58设置", "曲线59设置", "曲线60设置", "曲线61设置", "曲线62设置", "曲线63设置", "曲线64设置", "ID值", "数据模式"] ("DataInitDef")
                w1609 = "显控2" ("标题.文本")
                n1328 = event-data() -> ()  [unwired: 1 in, 8 out]
                n1329 = invoke on="控件配置文件" class="Tbl (严格)" method="Set Cell Value"("X Index"=1 ("X索引"), "Y Index"=w1608, "Value"="X" ("值")) -> ()  [unwired: 3 in, 6 out]
                n1330 = invoke on="控件配置文件" class="Tbl (严格)" method="Set Cell Value"("X Index"=0 ("X索引"), "Y Index"=w1608, "Value"=w1609) -> ()  [unwired: 3 in, 6 out]
                n1331 = property on="显控2" class="Str"("Caption.Text"=w1609) -> ()  [unwired: 2 in, 2 out]
                n1332 = property on="显控2设置" class="Str"("Val(Sgnl)"=w1609) -> ()  [unwired: 2 in, 2 out]
              }
              event "显控3": Shortcut Menu Selection (User) {
                w1613 = T9 12 items=["刷新间隔", "波特率", "布尔1设置项", "布尔2设置项", "布尔3设置项", "布尔4设置项", "布尔5设置项", "布尔6设置项", "布尔7设置项", "布尔8设置项", "显控1设置", "显控2设置", "显控3设置", "显控4设置", "显控5设置", "显控6设置", "显控7设置", "显控8设置", "显控9设置", "显控10设置", "显控11设置", "显控12设置", "设控1设置", "设控2设置", "设控3设置", "设控4设置", "设控5设置", "设控6设置", "设控7设置", "设控8设置", "曲线1设置", "曲线2设置", "曲线3设置", "曲线4设置", "曲线5设置", "曲线6设置", "曲线7设置", "曲线8设置", "曲线9设置", "曲线10设置", "曲线11设置", "曲线12设置", "曲线13设置", "曲线14设置", "曲线15设置", "曲线16设置", "曲线17设置", "曲线18设置", "曲线19设置", "曲线20设置", "曲线21设置", "曲线22设置", "曲线23设置", "曲线24设置", "曲线25设置", "曲线26设置", "曲线27设置", "曲线28设置", "曲线29设置", "曲线30设置", "曲线31设置", "曲线32设置", "曲线33设置", "曲线34设置", "曲线35设置", "曲线36设置", "曲线37设置", "曲线38设置", "曲线39设置", "曲线40设置", "曲线41设置", "曲线42设置", "曲线43设置", "曲线44设置", "曲线45设置", "曲线46设置", "曲线47设置", "曲线48设置", "曲线49设置", "曲线50设置", "曲线51设置", "曲线52设置", "曲线53设置", "曲线54设置", "曲线55设置", "曲线56设置", "曲线57设置", "曲线58设置", "曲线59设置", "曲线60设置", "曲线61设置", "曲线62设置", "曲线63设置", "曲线64设置", "ID值", "数据模式"] ("DataInitDef")
                w1614 = "显控3" ("标题.文本")
                n1333 = event-data() -> ()  [unwired: 1 in, 8 out]
                n1334 = invoke on="控件配置文件" class="Tbl (严格)" method="Set Cell Value"("X Index"=1 ("X索引"), "Y Index"=w1613, "Value"="X" ("值")) -> ()  [unwired: 3 in, 6 out]
                n1335 = invoke on="控件配置文件" class="Tbl (严格)" method="Set Cell Value"("X Index"=0 ("X索引"), "Y Index"=w1613, "Value"=w1614) -> ()  [unwired: 3 in, 6 out]
                n1336 = property on="显控3" class="Str"("Caption.Text"=w1614) -> ()  [unwired: 2 in, 2 out]
                n1337 = property on="显控3设置" class="Str"("Val(Sgnl)"=w1614) -> ()  [unwired: 2 in, 2 out]
              }
              event "显控4": Shortcut Menu Selection (User) {
                w1618 = T9 13 items=["刷新间隔", "波特率", "布尔1设置项", "布尔2设置项", "布尔3设置项", "布尔4设置项", "布尔5设置项", "布尔6设置项", "布尔7设置项", "布尔8设置项", "显控1设置", "显控2设置", "显控3设置", "显控4设置", "显控5设置", "显控6设置", "显控7设置", "显控8设置", "显控9设置", "显控10设置", "显控11设置", "显控12设置", "设控1设置", "设控2设置", "设控3设置", "设控4设置", "设控5设置", "设控6设置", "设控7设置", "设控8设置", "曲线1设置", "曲线2设置", "曲线3设置", "曲线4设置", "曲线5设置", "曲线6设置", "曲线7设置", "曲线8设置", "曲线9设置", "曲线10设置", "曲线11设置", "曲线12设置", "曲线13设置", "曲线14设置", "曲线15设置", "曲线16设置", "曲线17设置", "曲线18设置", "曲线19设置", "曲线20设置", "曲线21设置", "曲线22设置", "曲线23设置", "曲线24设置", "曲线25设置", "曲线26设置", "曲线27设置", "曲线28设置", "曲线29设置", "曲线30设置", "曲线31设置", "曲线32设置", "曲线33设置", "曲线34设置", "曲线35设置", "曲线36设置", "曲线37设置", "曲线38设置", "曲线39设置", "曲线40设置", "曲线41设置", "曲线42设置", "曲线43设置", "曲线44设置", "曲线45设置", "曲线46设置", "曲线47设置", "曲线48设置", "曲线49设置", "曲线50设置", "曲线51设置", "曲线52设置", "曲线53设置", "曲线54设置", "曲线55设置", "曲线56设置", "曲线57设置", "曲线58设置", "曲线59设置", "曲线60设置", "曲线61设置", "曲线62设置", "曲线63设置", "曲线64设置", "ID值", "数据模式"] ("DataInitDef")
                w1619 = "显控4" ("标题.文本")
                n1338 = event-data() -> ()  [unwired: 1 in, 8 out]
                n1339 = invoke on="控件配置文件" class="Tbl (严格)" method="Set Cell Value"("X Index"=1 ("X索引"), "Y Index"=w1618, "Value"="X" ("值")) -> ()  [unwired: 3 in, 6 out]
                n1340 = invoke on="控件配置文件" class="Tbl (严格)" method="Set Cell Value"("X Index"=0 ("X索引"), "Y Index"=w1618, "Value"=w1619) -> ()  [unwired: 3 in, 6 out]
                n1341 = property on="显控4" class="Str"("Caption.Text"=w1619) -> ()  [unwired: 2 in, 2 out]
                n1342 = property on="显控4设置" class="Str"("Val(Sgnl)"=w1619) -> ()  [unwired: 2 in, 2 out]
              }
              event "显控5": Shortcut Menu Selection (User) {
                w1623 = T9 14 items=["刷新间隔", "波特率", "布尔1设置项", "布尔2设置项", "布尔3设置项", "布尔4设置项", "布尔5设置项", "布尔6设置项", "布尔7设置项", "布尔8设置项", "显控1设置", "显控2设置", "显控3设置", "显控4设置", "显控5设置", "显控6设置", "显控7设置", "显控8设置", "显控9设置", "显控10设置", "显控11设置", "显控12设置", "设控1设置", "设控2设置", "设控3设置", "设控4设置", "设控5设置", "设控6设置", "设控7设置", "设控8设置", "曲线1设置", "曲线2设置", "曲线3设置", "曲线4设置", "曲线5设置", "曲线6设置", "曲线7设置", "曲线8设置", "曲线9设置", "曲线10设置", "曲线11设置", "曲线12设置", "曲线13设置", "曲线14设置", "曲线15设置", "曲线16设置", "曲线17设置", "曲线18设置", "曲线19设置", "曲线20设置", "曲线21设置", "曲线22设置", "曲线23设置", "曲线24设置", "曲线25设置", "曲线26设置", "曲线27设置", "曲线28设置", "曲线29设置", "曲线30设置", "曲线31设置", "曲线32设置", "曲线33设置", "曲线34设置", "曲线35设置", "曲线36设置", "曲线37设置", "曲线38设置", "曲线39设置", "曲线40设置", "曲线41设置", "曲线42设置", "曲线43设置", "曲线44设置", "曲线45设置", "曲线46设置", "曲线47设置", "曲线48设置", "曲线49设置", "曲线50设置", "曲线51设置", "曲线52设置", "曲线53设置", "曲线54设置", "曲线55设置", "曲线56设置", "曲线57设置", "曲线58设置", "曲线59设置", "曲线60设置", "曲线61设置", "曲线62设置", "曲线63设置", "曲线64设置", "ID值", "数据模式"] ("DataInitDef")
                w1624 = "显控5" ("标题.文本")
                n1343 = event-data() -> ()  [unwired: 1 in, 8 out]
                n1344 = invoke on="控件配置文件" class="Tbl (严格)" method="Set Cell Value"("X Index"=1 ("X索引"), "Y Index"=w1623, "Value"="X" ("值")) -> ()  [unwired: 3 in, 6 out]
                n1345 = invoke on="控件配置文件" class="Tbl (严格)" method="Set Cell Value"("X Index"=0 ("X索引"), "Y Index"=w1623, "Value"=w1624) -> ()  [unwired: 3 in, 6 out]
                n1346 = property on="显控5" class="Str"("Caption.Text"=w1624) -> ()  [unwired: 2 in, 2 out]
                n1347 = property on="显控5设置" class="Str"("Val(Sgnl)"=w1624) -> ()  [unwired: 2 in, 2 out]
              }
              event "显控6": Shortcut Menu Selection (User) {
                w1628 = T9 15 items=["刷新间隔", "波特率", "布尔1设置项", "布尔2设置项", "布尔3设置项", "布尔4设置项", "布尔5设置项", "布尔6设置项", "布尔7设置项", "布尔8设置项", "显控1设置", "显控2设置", "显控3设置", "显控4设置", "显控5设置", "显控6设置", "显控7设置", "显控8设置", "显控9设置", "显控10设置", "显控11设置", "显控12设置", "设控1设置", "设控2设置", "设控3设置", "设控4设置", "设控5设置", "设控6设置", "设控7设置", "设控8设置", "曲线1设置", "曲线2设置", "曲线3设置", "曲线4设置", "曲线5设置", "曲线6设置", "曲线7设置", "曲线8设置", "曲线9设置", "曲线10设置", "曲线11设置", "曲线12设置", "曲线13设置", "曲线14设置", "曲线15设置", "曲线16设置", "曲线17设置", "曲线18设置", "曲线19设置", "曲线20设置", "曲线21设置", "曲线22设置", "曲线23设置", "曲线24设置", "曲线25设置", "曲线26设置", "曲线27设置", "曲线28设置", "曲线29设置", "曲线30设置", "曲线31设置", "曲线32设置", "曲线33设置", "曲线34设置", "曲线35设置", "曲线36设置", "曲线37设置", "曲线38设置", "曲线39设置", "曲线40设置", "曲线41设置", "曲线42设置", "曲线43设置", "曲线44设置", "曲线45设置", "曲线46设置", "曲线47设置", "曲线48设置", "曲线49设置", "曲线50设置", "曲线51设置", "曲线52设置", "曲线53设置", "曲线54设置", "曲线55设置", "曲线56设置", "曲线57设置", "曲线58设置", "曲线59设置", "曲线60设置", "曲线61设置", "曲线62设置", "曲线63设置", "曲线64设置", "ID值", "数据模式"] ("DataInitDef")
                w1629 = "显控6" ("标题.文本")
                n1348 = event-data() -> ()  [unwired: 1 in, 8 out]
                n1349 = invoke on="控件配置文件" class="Tbl (严格)" method="Set Cell Value"("X Index"=1 ("X索引"), "Y Index"=w1628, "Value"="X" ("值")) -> ()  [unwired: 3 in, 6 out]
                n1350 = invoke on="控件配置文件" class="Tbl (严格)" method="Set Cell Value"("X Index"=0 ("X索引"), "Y Index"=w1628, "Value"=w1629) -> ()  [unwired: 3 in, 6 out]
                n1351 = property on="显控6" class="Str"("Caption.Text"=w1629) -> ()  [unwired: 2 in, 2 out]
                n1352 = property on="显控6设置" class="Str"("Val(Sgnl)"=w1629) -> ()  [unwired: 2 in, 2 out]
              }
              event "显控7": Shortcut Menu Selection (User) {
                w1633 = T9 16 items=["刷新间隔", "波特率", "布尔1设置项", "布尔2设置项", "布尔3设置项", "布尔4设置项", "布尔5设置项", "布尔6设置项", "布尔7设置项", "布尔8设置项", "显控1设置", "显控2设置", "显控3设置", "显控4设置", "显控5设置", "显控6设置", "显控7设置", "显控8设置", "显控9设置", "显控10设置", "显控11设置", "显控12设置", "设控1设置", "设控2设置", "设控3设置", "设控4设置", "设控5设置", "设控6设置", "设控7设置", "设控8设置", "曲线1设置", "曲线2设置", "曲线3设置", "曲线4设置", "曲线5设置", "曲线6设置", "曲线7设置", "曲线8设置", "曲线9设置", "曲线10设置", "曲线11设置", "曲线12设置", "曲线13设置", "曲线14设置", "曲线15设置", "曲线16设置", "曲线17设置", "曲线18设置", "曲线19设置", "曲线20设置", "曲线21设置", "曲线22设置", "曲线23设置", "曲线24设置", "曲线25设置", "曲线26设置", "曲线27设置", "曲线28设置", "曲线29设置", "曲线30设置", "曲线31设置", "曲线32设置", "曲线33设置", "曲线34设置", "曲线35设置", "曲线36设置", "曲线37设置", "曲线38设置", "曲线39设置", "曲线40设置", "曲线41设置", "曲线42设置", "曲线43设置", "曲线44设置", "曲线45设置", "曲线46设置", "曲线47设置", "曲线48设置", "曲线49设置", "曲线50设置", "曲线51设置", "曲线52设置", "曲线53设置", "曲线54设置", "曲线55设置", "曲线56设置", "曲线57设置", "曲线58设置", "曲线59设置", "曲线60设置", "曲线61设置", "曲线62设置", "曲线63设置", "曲线64设置", "ID值", "数据模式"] ("DataInitDef")
                w1634 = "显控7" ("标题.文本")
                n1353 = event-data() -> ()  [unwired: 1 in, 8 out]
                n1354 = invoke on="控件配置文件" class="Tbl (严格)" method="Set Cell Value"("X Index"=1 ("X索引"), "Y Index"=w1633, "Value"="X" ("值")) -> ()  [unwired: 3 in, 6 out]
                n1355 = invoke on="控件配置文件" class="Tbl (严格)" method="Set Cell Value"("X Index"=0 ("X索引"), "Y Index"=w1633, "Value"=w1634) -> ()  [unwired: 3 in, 6 out]
                n1356 = property on="显控7" class="Str"("Caption.Text"=w1634) -> ()  [unwired: 2 in, 2 out]
                n1357 = property on="显控7设置" class="Str"("Val(Sgnl)"=w1634) -> ()  [unwired: 2 in, 2 out]
              }
              event "显控8": Shortcut Menu Selection (User) {
                w1638 = T9 17 items=["刷新间隔", "波特率", "布尔1设置项", "布尔2设置项", "布尔3设置项", "布尔4设置项", "布尔5设置项", "布尔6设置项", "布尔7设置项", "布尔8设置项", "显控1设置", "显控2设置", "显控3设置", "显控4设置", "显控5设置", "显控6设置", "显控7设置", "显控8设置", "显控9设置", "显控10设置", "显控11设置", "显控12设置", "设控1设置", "设控2设置", "设控3设置", "设控4设置", "设控5设置", "设控6设置", "设控7设置", "设控8设置", "曲线1设置", "曲线2设置", "曲线3设置", "曲线4设置", "曲线5设置", "曲线6设置", "曲线7设置", "曲线8设置", "曲线9设置", "曲线10设置", "曲线11设置", "曲线12设置", "曲线13设置", "曲线14设置", "曲线15设置", "曲线16设置", "曲线17设置", "曲线18设置", "曲线19设置", "曲线20设置", "曲线21设置", "曲线22设置", "曲线23设置", "曲线24设置", "曲线25设置", "曲线26设置", "曲线27设置", "曲线28设置", "曲线29设置", "曲线30设置", "曲线31设置", "曲线32设置", "曲线33设置", "曲线34设置", "曲线35设置", "曲线36设置", "曲线37设置", "曲线38设置", "曲线39设置", "曲线40设置", "曲线41设置", "曲线42设置", "曲线43设置", "曲线44设置", "曲线45设置", "曲线46设置", "曲线47设置", "曲线48设置", "曲线49设置", "曲线50设置", "曲线51设置", "曲线52设置", "曲线53设置", "曲线54设置", "曲线55设置", "曲线56设置", "曲线57设置", "曲线58设置", "曲线59设置", "曲线60设置", "曲线61设置", "曲线62设置", "曲线63设置", "曲线64设置", "ID值", "数据模式"] ("DataInitDef")
                w1639 = "显控8" ("标题.文本")
                n1358 = event-data() -> ()  [unwired: 1 in, 8 out]
                n1359 = invoke on="控件配置文件" class="Tbl (严格)" method="Set Cell Value"("X Index"=1 ("X索引"), "Y Index"=w1638, "Value"="X" ("值")) -> ()  [unwired: 3 in, 6 out]
                n1360 = invoke on="控件配置文件" class="Tbl (严格)" method="Set Cell Value"("X Index"=0 ("X索引"), "Y Index"=w1638, "Value"=w1639) -> ()  [unwired: 3 in, 6 out]
                n1361 = property on="显控8" class="Str"("Caption.Text"=w1639) -> ()  [unwired: 2 in, 2 out]
                n1362 = property on="显控8设置" class="Str"("Val(Sgnl)"=w1639) -> ()  [unwired: 2 in, 2 out]
              }
              event "显控9": Shortcut Menu Selection (User) {
                w1643 = T9 18 items=["刷新间隔", "波特率", "布尔1设置项", "布尔2设置项", "布尔3设置项", "布尔4设置项", "布尔5设置项", "布尔6设置项", "布尔7设置项", "布尔8设置项", "显控1设置", "显控2设置", "显控3设置", "显控4设置", "显控5设置", "显控6设置", "显控7设置", "显控8设置", "显控9设置", "显控10设置", "显控11设置", "显控12设置", "设控1设置", "设控2设置", "设控3设置", "设控4设置", "设控5设置", "设控6设置", "设控7设置", "设控8设置", "曲线1设置", "曲线2设置", "曲线3设置", "曲线4设置", "曲线5设置", "曲线6设置", "曲线7设置", "曲线8设置", "曲线9设置", "曲线10设置", "曲线11设置", "曲线12设置", "曲线13设置", "曲线14设置", "曲线15设置", "曲线16设置", "曲线17设置", "曲线18设置", "曲线19设置", "曲线20设置", "曲线21设置", "曲线22设置", "曲线23设置", "曲线24设置", "曲线25设置", "曲线26设置", "曲线27设置", "曲线28设置", "曲线29设置", "曲线30设置", "曲线31设置", "曲线32设置", "曲线33设置", "曲线34设置", "曲线35设置", "曲线36设置", "曲线37设置", "曲线38设置", "曲线39设置", "曲线40设置", "曲线41设置", "曲线42设置", "曲线43设置", "曲线44设置", "曲线45设置", "曲线46设置", "曲线47设置", "曲线48设置", "曲线49设置", "曲线50设置", "曲线51设置", "曲线52设置", "曲线53设置", "曲线54设置", "曲线55设置", "曲线56设置", "曲线57设置", "曲线58设置", "曲线59设置", "曲线60设置", "曲线61设置", "曲线62设置", "曲线63设置", "曲线64设置", "ID值", "数据模式"] ("DataInitDef")
                w1644 = "显控9" ("标题.文本")
                n1363 = event-data() -> ()  [unwired: 1 in, 8 out]
                n1364 = invoke on="控件配置文件" class="Tbl (严格)" method="Set Cell Value"("X Index"=1 ("X索引"), "Y Index"=w1643, "Value"="X" ("值")) -> ()  [unwired: 3 in, 6 out]
                n1365 = invoke on="控件配置文件" class="Tbl (严格)" method="Set Cell Value"("X Index"=0 ("X索引"), "Y Index"=w1643, "Value"=w1644) -> ()  [unwired: 3 in, 6 out]
                n1366 = property on="显控9" class="Str"("Caption.Text"=w1644) -> ()  [unwired: 2 in, 2 out]
                n1367 = property on="显控9设置" class="Str"("Val(Sgnl)"=w1644) -> ()  [unwired: 2 in, 2 out]
              }
              event "显控10": Shortcut Menu Selection (User) {
                w1648 = T9 19 items=["刷新间隔", "波特率", "布尔1设置项", "布尔2设置项", "布尔3设置项", "布尔4设置项", "布尔5设置项", "布尔6设置项", "布尔7设置项", "布尔8设置项", "显控1设置", "显控2设置", "显控3设置", "显控4设置", "显控5设置", "显控6设置", "显控7设置", "显控8设置", "显控9设置", "显控10设置", "显控11设置", "显控12设置", "设控1设置", "设控2设置", "设控3设置", "设控4设置", "设控5设置", "设控6设置", "设控7设置", "设控8设置", "曲线1设置", "曲线2设置", "曲线3设置", "曲线4设置", "曲线5设置", "曲线6设置", "曲线7设置", "曲线8设置", "曲线9设置", "曲线10设置", "曲线11设置", "曲线12设置", "曲线13设置", "曲线14设置", "曲线15设置", "曲线16设置", "曲线17设置", "曲线18设置", "曲线19设置", "曲线20设置", "曲线21设置", "曲线22设置", "曲线23设置", "曲线24设置", "曲线25设置", "曲线26设置", "曲线27设置", "曲线28设置", "曲线29设置", "曲线30设置", "曲线31设置", "曲线32设置", "曲线33设置", "曲线34设置", "曲线35设置", "曲线36设置", "曲线37设置", "曲线38设置", "曲线39设置", "曲线40设置", "曲线41设置", "曲线42设置", "曲线43设置", "曲线44设置", "曲线45设置", "曲线46设置", "曲线47设置", "曲线48设置", "曲线49设置", "曲线50设置", "曲线51设置", "曲线52设置", "曲线53设置", "曲线54设置", "曲线55设置", "曲线56设置", "曲线57设置", "曲线58设置", "曲线59设置", "曲线60设置", "曲线61设置", "曲线62设置", "曲线63设置", "曲线64设置", "ID值", "数据模式"] ("DataInitDef")
                w1649 = "显控10" ("标题.文本")
                n1368 = event-data() -> ()  [unwired: 1 in, 8 out]
                n1369 = invoke on="控件配置文件" class="Tbl (严格)" method="Set Cell Value"("X Index"=1 ("X索引"), "Y Index"=w1648, "Value"="X" ("值")) -> ()  [unwired: 3 in, 6 out]
                n1370 = invoke on="控件配置文件" class="Tbl (严格)" method="Set Cell Value"("X Index"=0 ("X索引"), "Y Index"=w1648, "Value"=w1649) -> ()  [unwired: 3 in, 6 out]
                n1371 = property on="显控10" class="Str"("Caption.Text"=w1649) -> ()  [unwired: 2 in, 2 out]
                n1372 = property on="显控10设置" class="Str"("Val(Sgnl)"=w1649) -> ()  [unwired: 2 in, 2 out]
              }
              event "显控11": Shortcut Menu Selection (User) {
                w1653 = T9 20 items=["刷新间隔", "波特率", "布尔1设置项", "布尔2设置项", "布尔3设置项", "布尔4设置项", "布尔5设置项", "布尔6设置项", "布尔7设置项", "布尔8设置项", "显控1设置", "显控2设置", "显控3设置", "显控4设置", "显控5设置", "显控6设置", "显控7设置", "显控8设置", "显控9设置", "显控10设置", "显控11设置", "显控12设置", "设控1设置", "设控2设置", "设控3设置", "设控4设置", "设控5设置", "设控6设置", "设控7设置", "设控8设置", "曲线1设置", "曲线2设置", "曲线3设置", "曲线4设置", "曲线5设置", "曲线6设置", "曲线7设置", "曲线8设置", "曲线9设置", "曲线10设置", "曲线11设置", "曲线12设置", "曲线13设置", "曲线14设置", "曲线15设置", "曲线16设置", "曲线17设置", "曲线18设置", "曲线19设置", "曲线20设置", "曲线21设置", "曲线22设置", "曲线23设置", "曲线24设置", "曲线25设置", "曲线26设置", "曲线27设置", "曲线28设置", "曲线29设置", "曲线30设置", "曲线31设置", "曲线32设置", "曲线33设置", "曲线34设置", "曲线35设置", "曲线36设置", "曲线37设置", "曲线38设置", "曲线39设置", "曲线40设置", "曲线41设置", "曲线42设置", "曲线43设置", "曲线44设置", "曲线45设置", "曲线46设置", "曲线47设置", "曲线48设置", "曲线49设置", "曲线50设置", "曲线51设置", "曲线52设置", "曲线53设置", "曲线54设置", "曲线55设置", "曲线56设置", "曲线57设置", "曲线58设置", "曲线59设置", "曲线60设置", "曲线61设置", "曲线62设置", "曲线63设置", "曲线64设置", "ID值", "数据模式"] ("DataInitDef")
                w1654 = "显控11" ("标题.文本")
                n1373 = event-data() -> ()  [unwired: 1 in, 8 out]
                n1374 = invoke on="控件配置文件" class="Tbl (严格)" method="Set Cell Value"("X Index"=1 ("X索引"), "Y Index"=w1653, "Value"="X" ("值")) -> ()  [unwired: 3 in, 6 out]
                n1375 = invoke on="控件配置文件" class="Tbl (严格)" method="Set Cell Value"("X Index"=0 ("X索引"), "Y Index"=w1653, "Value"=w1654) -> ()  [unwired: 3 in, 6 out]
                n1376 = property on="显控11" class="Str"("Caption.Text"=w1654) -> ()  [unwired: 2 in, 2 out]
                n1377 = property on="显控11设置" class="Str"("Val(Sgnl)"=w1654) -> ()  [unwired: 2 in, 2 out]
              }
              event "显控12": Shortcut Menu Selection (User) {
